vi "Control Panel (No Objects).vi"(8 "error in":errorcluster, 10 "Set Voltage":dbl=150.0 min=0.0 max=700.0, 11 "VISA Resource Name":refnum<visa-resource-name>="USB0::0x0699::0x036A::C035909::INSTR") -> (0 "error out":errorcluster, 2 "Actual Voltage":dbl, 3 "VISA resource name out":refnum<visa-resource-name>)   [LabVIEW 2023]
uses:
  Tektronix TDS 2024B Oscilloscope/Tektronix TDS 200 1000 2000 Series/Tektronix TDS 200 1000 2000 Series.lvlib
panel:
  out "Actual Voltage":dbl(slide) scale=0.0..500.0
  out "Set Voltage":dbl(slide) scale=0.6..500.0
  out "At Voltage":bool
  out "Waveform Data":waveform(dbl)(graph)
  in  "Output Terminal":tag="/Dev2/PFI8"
  in  "Counter":tag="Dev2/ctr0"
  in  "Stop":bool
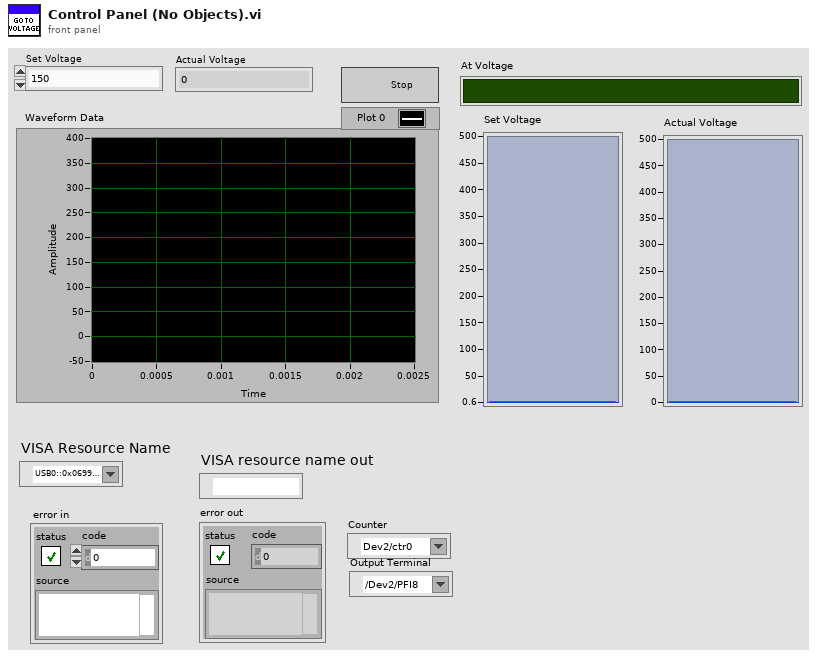
[diagram p1: front panel]
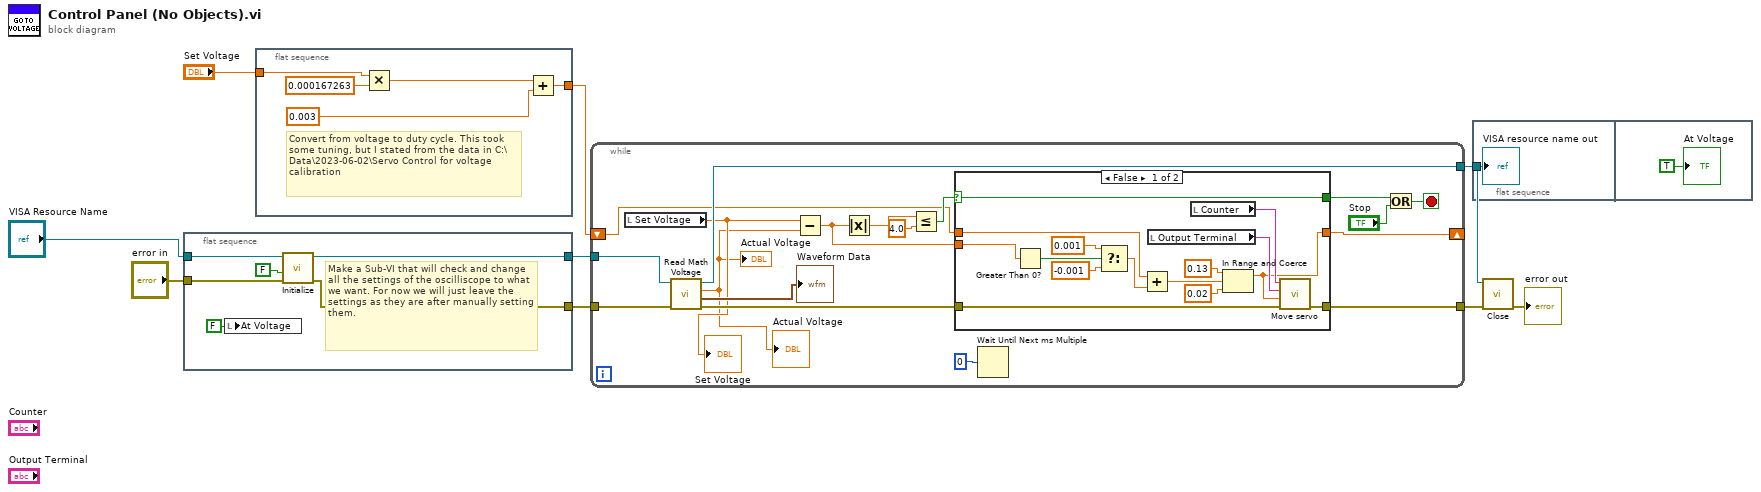
[diagram p0: block diagram]
diagram:
  n1 = flat-sequence {
    tunnel: [w15] -> w9
    tunnel: [w14] -> w8
    tunnel: "error in" -> [w12]
    tunnel: "VISA Resource Name" -> [w11]
    frame #0 {
      # "Make a Sub-VI that will check and change all the settings of the oscilliscope to what we want. For now we will just leave the settings as they are after manually setting them."
      n2 = local write "At Voltage"(FALSE ("Boolean")) -> ()
      n3 = call "Initialize.vi"("error in (no error)"=w12, "Reset? (T: Yes)"=FALSE, "VISA resource name"=w11) -> ("error out"=w15:errorcluster, "VISA resource name out"=w14:refnum<visa-resource-name>)  [unwired: 7 in]
    }
  }
  n4 = flat-sequence {
    tunnel: "Set Voltage" -> [w20]
    tunnel: [w16] -> w2
    frame #0 {
      # "Convert from voltage to duty cycle. This took some tuning, but I stated from the data in C:\\Data\\2023-06-02\\Servo Control for voltage calibration"
      n5 = Multiply(x=w20, y=0.000167263) -> (x*y=w19:dbl)
      n6 = Add(x=w19, y=0.003) -> (x+y=w16:dbl)
    }
  }
  n7 = while {
    tunnel: w9 -> [w35]
    tunnel: w8 -> [w34]
    tunnel: [w33] -> w4
    tunnel: [w30] -> w3
    shift-right: [w26] -> _
    shift-left: w2 -> [w25]
    stop <- w29 stop-if-true
    n8 = local read "Set Voltage"() -> (w22:dbl)
    "Set Voltage" <- w22
    n9 = call "Read Math Voltage.vi"("error in (no error)"=w35, "VISA resource name"=w34) -> ("error out"=w31:errorcluster, "Waveform Data"=→"Waveform Data":waveform(dbl), "amplitude"=w21:dbl, "VISA resource name out"=w33:refnum<visa-resource-name>)  [unwired: 6 in]
    "Actual Voltage" <- w21
    "Actual Voltage" <- w21
    n10 = Subtract(x=w22, y=w21) -> (x-y=w24:dbl)
    n11 = Absolute Value(x=w24) -> (abs(x)=w37:dbl)
    n12 = Less Or Equal?(x=w37, y=4.0) -> (x <= y?=w32:bool)
    n13 = case shown="False" w32 {
      selector: w32 -> [w49 w55]
      tunnel: w31 -> [w51 w56]
      tunnel: [w50 w56] -> w30
      tunnel: [w49 w55] -> w27
      tunnel: [w41 w54] -> w26
      tunnel: w25 -> [w43 w54]
      tunnel: w24 -> [w48 _]
      frame False {
        n14 = Greater Than 0?(x=w48) -> (x > 0?=w47:bool)
        n15 = Select(t=0.001, s=w47, f=-0.001) -> (s? t:f=w44:dbl)
        n16 = Add(x=w43, y=w44) -> (x+y=w42:dbl)
        n17 = local read "Output Terminal"() -> (w53:tag)
        n18 = local read "Counter"() -> (w52:tag)
        n19 = In Range and Coerce(upper limit=0.13, x=w42, lower limit=0.02) -> (coerced(x)=w41:dbl)  [unwired: 1 out]
        n20 = call "Move servo.vi"("error in"=w51, "Duty Cycle"=w41, "Output Terminal"=w53, "Counter"=w52) -> ("error out"=w50:errorcluster)  [unwired: 6 in, 1 out]
      }
      frame True {
      }
    }
    n21 = Wait Until Next ms Multiple(millisecond multiple=u32 0) -> ()  [unwired: 1 out]
    n22 = Or(x=w27, y="Stop") -> (x .or. y?=w29:bool)
  }
  n23 = flat-sequence {
    tunnel: w4 -> [w57]
    frame #0 {
      "VISA resource name out" <- w57
    }
    frame #1 {
      "At Voltage" <- TRUE ("Boolean")
    }
  }
  n24 = call "Close.vi"("error in (no error)"=w3, "VISA resource name"=w4) -> ("error out"=→"error out":errorcluster)  [unwired: 9 out]
